vi "FocusOnThisItem.vi"(8 "error in (no error)":errorcluster, 9 "Focus?(False)":bool, 10 "ItemCtlRef":refnum<vi>, 11 "MakeTableItem in":refnum<class "ConcreteTableItem.lvclass">) -> (0 "error out":errorcluster, 3 "MakeTableItem out":refnum<class "ConcreteTableItem.lvclass">)   [LabVIEW 2015, in "ActorManagement.lvlib" / "ConcreteTableItem.lvclass"]
uses:
  ConcreteTableItem.lvclass
  ConcreteTableItem.lvclass/ConcreteTableItem.ctl
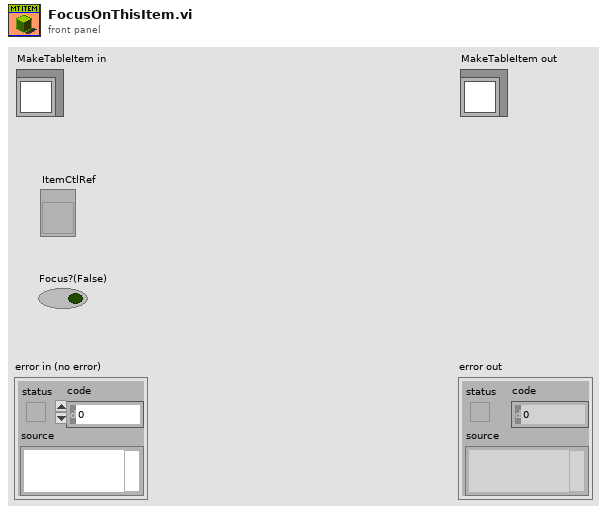
[diagram p1: front panel]
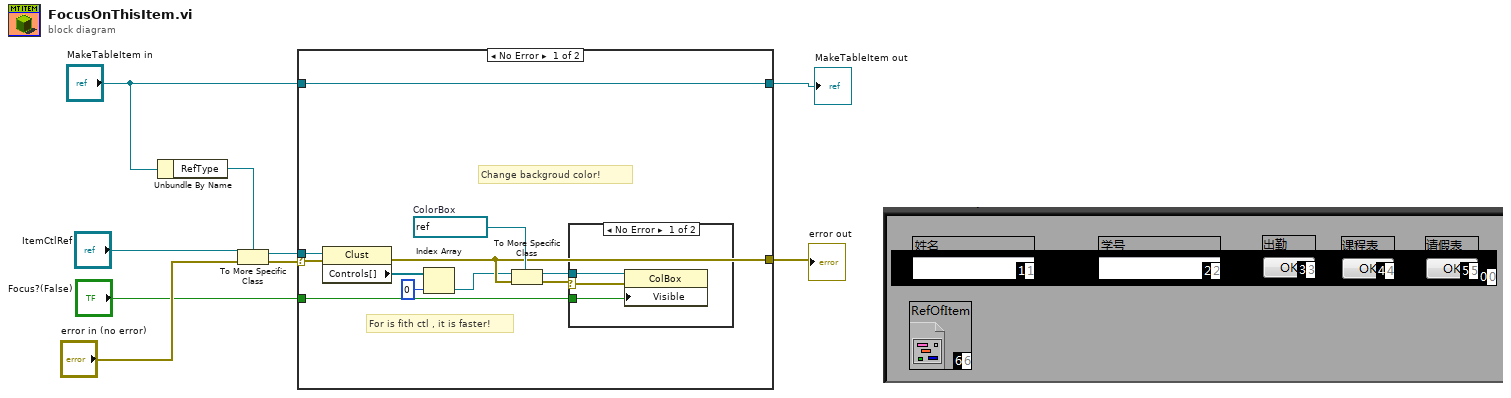
[diagram p0: block diagram]
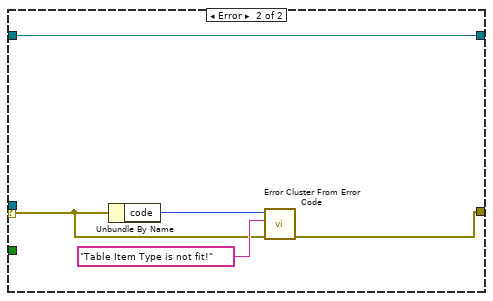
[diagram p3: hidden frame]
diagram:
  n1 = Unbundle By Name("MakeTableItem in") -> ("RefType"=w8:refnum<vi>)
  n2 = To More Specific Class(target class=w8, reference="ItemCtlRef", error in="error in (no error)") -> (specific class reference=w5:refnum<vi>, error out=w6:errorcluster)
  n3 = case shown="No Error" w6 {
    selector: w6 -> [w19 w25]
    tunnel: w5 -> [w20 _]
    tunnel: "MakeTableItem in" -> [w16 w28]
    tunnel: [w17 w24] -> w3
    tunnel: [w16 w28] -> w2
    tunnel: "Focus?(False)" -> [w15 _]
    frame No Error {
      w18 = refnum<vi> refnum  # ColorBox
      # "For is fith ctl , it is faster!"
      # "Change backgroud color!"
      n4 = property class="Clust"(reference=w20, error in=w19) -> (error out=w17:errorcluster, "Controls[]"=w12:refnum<vi>[])  [unwired: 1 out]
      n5 = Index Array(array=w12, index=0) -> (element=w10:refnum<vi>)
      n6 = To More Specific Class(target class=w18, reference=w10, error in=w17) -> (specific class reference=w13:refnum<vi>, error out=w14:errorcluster)
      n7 = case shown="No Error" w14 {
        selector: w14 -> [w23 _]
        tunnel: w13 -> [w22 _]
        tunnel: w15 -> [w21 _]
        frame No Error {
          n8 = property class="ColBox"(reference=w22, error in=w23, "Visible"=w21) -> ()  [unwired: 2 out]
        }
        frame Error {
        }
      }
    }
    frame Error {
      n9 = Unbundle By Name(w25) -> ("code"=w27:i32)
      n10 = call <vilib>:"Error Cluster From Error Code.vi"("error in (no error)"=w25, "error message (\"\")"="Table Item Type is not fit!" ("error message (\"\")"), "error code (0)"=w27) -> ("error out"=w24:errorcluster)  [unwired: 6 in]
    }
  }
  "error out" <- w3
  "MakeTableItem out" <- w2
